vi "Parse.vi"(8 "Error In":errorcluster, 11 "Parser In":refnum<class "Parser.lvclass">) -> (0 "Error Out":errorcluster, 2 "Tokens":refnum<class "Abstract.lvclass">[](array[class]), 3 "Parser Out":refnum<class "Parser.lvclass">)   [LabVIEW 2018, in "Toolkit.lvlib" / "Parser.lvclass"]
uses:
  Parser.lvclass
  Tokens/Abstract/Abstract.lvclass
  Parser.lvclass/Parser.ctl
  Support/Is Open Delimiter.vi
  Support/Pop Content.vi
  Support/Has Content.vi
  Support/Add Text Token.vi
  Support/Peek Content.vi
  Support/Is Close Delimiter.vi
  Support/Tokenize Tag.vi
  Support/Ignore Comment.vi
  Support/Change Delimiters.vi
  Tokens/Text/Text.lvclass
  D:/Users/cfield/Code/Field R&D Services/Mustache/trunk/src/Mustache/Public/Tokens/Public/Abstract/Abstract.lvclass
  Tokens/EscapedVariable/EscapedVariable.lvclass
  D:/Users/cfield/Code/Field R&D Services/Mustache/trunk/src/Mustache/Public/Tokens/Public/Keyable/Keyable.lvclass
  Tokens/UnescapedVariable/UnescapedVariable.lvclass
  Tokens/BeginSection/BeginSection.lvclass
  Tokens/InvertedSection/InvertedSection.lvclass
  Tokens/EndSection/EndSection.lvclass
  Tokens/Partial/Partial.lvclass
  Tokens/Keyable/API/Keyable.lvclass
  Tokens/Text/API/New.vi
  <vilib>/Utility/error.llb/Trim Whitespace.vi
  Tokens/EscapedVariable/API/New.vi
  Tokens/UnescapedVariable/API/New.vi
  Tokens/BeginSection/API/New.vi
  Tokens/InvertedSection/API/New.vi
  Tokens/EndSection/API/New.vi
  Tokens/Partial/API/New.vi
  Readers/Abstract/Abstract.lvclass
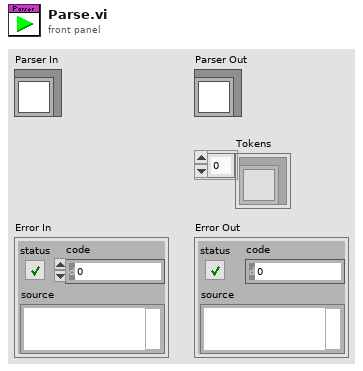
[diagram p1: front panel]
types:
  T1 = typedef "Toolkit.lvlib/Parser.lvclass/States.ctl" = enum16{"Text", "Open Delimiter", "Tag Type", "Tag Key", "Close Delimiter"}
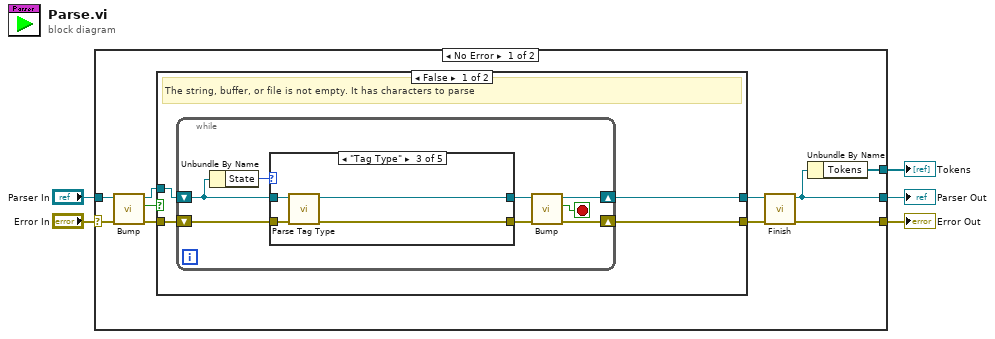
[diagram p0: block diagram]
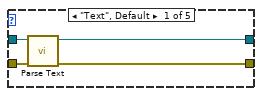
[diagram p2: hidden frame]
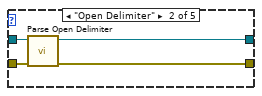
[diagram p3: hidden frame]
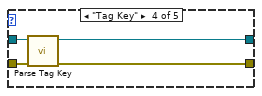
[diagram p4: hidden frame]
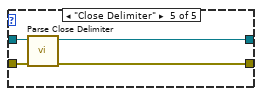
[diagram p5: hidden frame]
diagram:
  n1 = case shown="No Error" "Error In" {
    selector: "Error In" -> [w13 w51]
    tunnel: "Parser In" -> [w12 w50]
    tunnel: [w6 w51] -> w3
    tunnel: [w8 w50] -> w2
    tunnel: [w14 _] -> w1
    frame No Error {
      n2 = call "Bump.vi"("Error In"=w13, "Parser In"=w12) -> ("Error Out"=w10:errorcluster, "Done"=w9:bool, "Parser Out"=w11:refnum<class "Parser.lvclass">)  [unwired: 7 in]
      n3 = case shown="False" w9 {
        tunnel: [w17 w48] -> w7
        tunnel: [w16 w49] -> w15
        tunnel: w10 -> [w19 w48]
        tunnel: w11 -> [w18 w49]
        frame False {
          # "The string, buffer, or file is not empty. It has characters to parse"
          n4 = while {
            shift-right: [w21] -> w17
            shift-left: w19 -> [w25]
            shift-right: [w23] -> w16
            shift-left: w18 -> [w26]
            stop <- w22 stop-if-true
            n5 = Unbundle By Name(w26) -> ("State"=w27:T1)
            n6 = case shown="\"Tag Type\"" w27 {
              tunnel: w25 -> [w30 w35 w36 w40 w44]
              tunnel: w26 -> [w31 w34 w39 w43 w47]
              tunnel: [w29 w33 w38 w42 w46] -> w24
              tunnel: [w28 w32 w37 w41 w45] -> w20
              frame "Text", Default {
                n7 = call "Parse Text.vi"("Error In"=w30, "Parser In"=w31) -> ("Error Out"=w28:errorcluster, "Parser Out"=w29:refnum<class "Parser.lvclass">)  [unwired: 8 in]
              }
              frame "Open Delimiter" {
                n8 = call "Parse Open Delimiter.vi"("Error In"=w35, "Parser In"=w34) -> ("Error Out"=w32:errorcluster, "Parser Out"=w33:refnum<class "Parser.lvclass">)  [unwired: 8 in]
              }
              frame "Tag Type" {
                n9 = call "Parse Tag Type.vi"("Error In"=w36, "Parser In"=w39) -> ("Error Out"=w37:errorcluster, "Parser Out"=w38:refnum<class "Parser.lvclass">)  [unwired: 8 in]
              }
              frame "Tag Key" {
                n10 = call "Parse Tag Key.vi"("Error In"=w40, "Parser In"=w43) -> ("Error Out"=w41:errorcluster, "Parser Out"=w42:refnum<class "Parser.lvclass">)  [unwired: 8 in]
              }
              frame "Close Delimiter" {
                n11 = call "Parse Close Delimiter.vi"("Error In"=w44, "Parser In"=w47) -> ("Error Out"=w45:errorcluster, "Parser Out"=w46:refnum<class "Parser.lvclass">)  [unwired: 8 in]
              }
            }
            n12 = call "Bump.vi"("Error In"=w20, "Parser In"=w24) -> ("Error Out"=w21:errorcluster, "Done"=w22:bool, "Parser Out"=w23:refnum<class "Parser.lvclass">)  [unwired: 7 in]
          }
        }
        frame True {
          # "The string, buffer, file, etc. is empty. There is nothing to do."
        }
      }
      n13 = call "Finish.vi"("Error In"=w7, "Parser In"=w15) -> ("Error Out"=w6:errorcluster, "Parser Out"=w8:refnum<class "Parser.lvclass">)  [unwired: 8 in]
      n14 = Unbundle By Name(w8) -> ("Tokens"=w14:refnum<class "Abstract.lvclass">[])
    }
    frame Error {
    }
  }
  "Error Out" <- w3
  "Parser Out" <- w2
  "Tokens" <- w1
